vi "num2key (SubVI).vi"(10 "Img current":dbl, 11 "String in":string) -> (3 "String out":string)   [LabVIEW 2021]
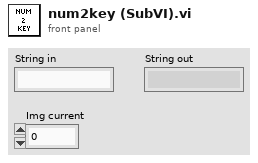
[diagram p1: front panel]
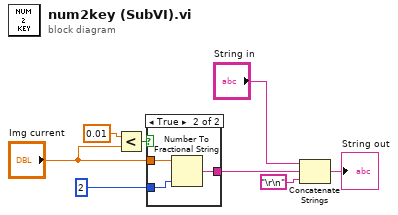
[diagram p0: block diagram]
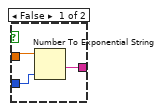
[diagram p2: hidden frame]
diagram:
  n1 = Less?(x=0.01, y="Img current") -> (x < y?=w4:bool)
  n2 = case shown="True" w4 {
    tunnel: "Img current" -> [w10 w14]
    tunnel: [w11 w13] -> w5
    tunnel: i16 2 ("precision (6)") -> [w9 w12]
    frame False {
      n3 = Number To Exponential String(number=w10, precision (6)=w9) -> (E-format string=w11:string)  [unwired: 2 in]
    }
    frame True {
      n4 = Number To Fractional String(number=w14, precision (6)=w12) -> (F-format string=w13:string)  [unwired: 2 in]
    }
  }
  n5 = Concatenate Strings("String in", w5, "\r\n") -> (→"String out":string)
